vi "SVXMPL_Snd Read Waveform.vi"(8 "error in (no error)":errorcluster, 11 "wave file path":path) -> (0 "error out":errorcluster, 2 "Channel 2":waveform(dbl), 3 "Channel 1":waveform(dbl), 4 "SVT Wav info":T1)   [LabVIEW 2017]
panel:
  in  "SVT Wav info":T1
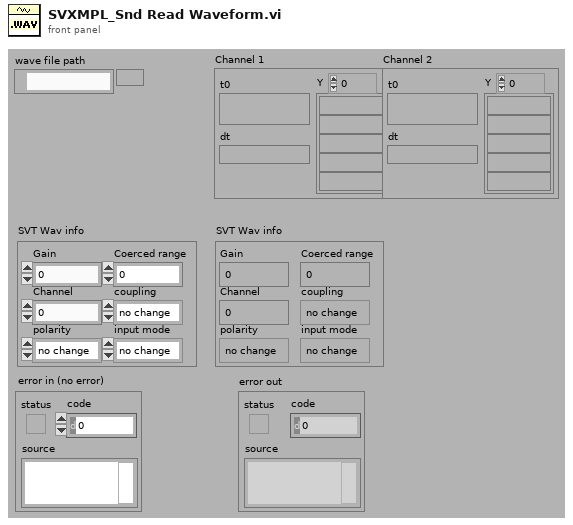
[diagram p1: front panel]
types:
  T1 = cluster{"Gain":u16, "Coerced range":u16, "Channel":u16, "coupling":enum16{"no change", "DC", "AC", "ground", "internal reference"}, "polarity":enum16{"no change", "bipolar", "unipolar"}, "input mode":enum16{"no change", "differential", "rse", "nrse"}}
  T2 = typedef "Sound Format.ctl" = cluster{"sound quality":enum16{"mono", "stereo"}, "rate":enum16{"11025", "22050", "44100", "8000"}, "bits per sample":enum16{"8 bit", "16 bit"}}
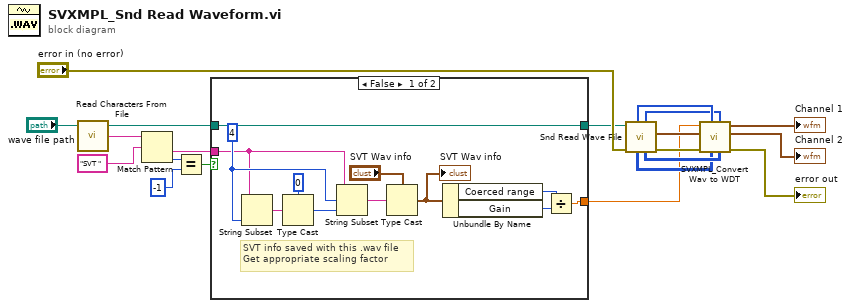
[diagram p0: block diagram]
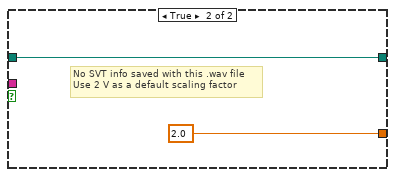
[diagram p2: hidden frame]
diagram:
  n1 = call <vilib>:"Read Characters From File.vi"("file path (dialog if empty)"="wave file path") -> ("new file path (NotAPath if cancelled)"=w5:path, "character string"=w9:string)  [unwired: 5 in, 2 out]
  n2 = Match Pattern(string=w9, regular expression="SVT ") -> (after substring=w2:string, offset past match=w7:i32)  [unwired: 1 in, 2 out]
  n3 = Equal?(x=w7, y=-1) -> (x = y?=w3:bool)
  n4 = case shown="False" w3 {
    tunnel: w5 -> [w32 w34]
    tunnel: [w32 w34] -> w4
    tunnel: w2 -> [w28 _]
    tunnel: [w23 2.0] -> w1
    frame False {
      w31 = 4 ("length (rest)")
      (unwired) 4 ("Array Length")
      # "SVT info saved with this .wav file\nGet appropriate scaling factor"
      n5 = String Subset(string=w28, length (rest)=w31) -> (substring=w30:string)  [unwired: 1 in]
      n6 = Type Cast(type=u32 0, x=w30) -> (*(type *) &x=w27:u32)
      n7 = String Subset(string=w28, offset (0)=w31, length (rest)=w27) -> (substring=w25:string)
      n8 = Type Cast(type="SVT Wav info", x=w25) -> (*(type *) &x=w24:T1)
      "SVT Wav info" <- w24
      n9 = Unbundle By Name(w24) -> ("Coerced range"=w22:u16, "Gain"=w21:u16)
      n10 = Divide(x=w22, y=w21) -> (x/y=w23:dbl)
    }
    frame True {
      # "No SVT info saved with this .wav file\nUse 2 V as a default scaling factor"
    }
  }
  n11 = call <vilib>:"Snd Read Wave File.vi"("error in (no error)"="error in (no error)", "wave file path"=w4) -> ("error out"=w20:errorcluster, "sound format"=w19:T2, "stereo 16-bit"=w15:i16[][], "mono 16-bit"=w17:i16[], "stereo 8-bit"=w14:u8[][], "mono 8-bit"=w18:u8[])  [unwired: 3 in, 1 out]
  n12 = call <vilib>:"SVXMPL_Convert Wav to WDT.vi"("stereo 16-bit"=w15, "mono 16-bit"=w17, "stereo 8-bit"=w14, "mono 8-bit"=w18, "error in (no error)"=w20, "sound format"=w19, "Gain"=w1) -> ("error out"=→"error out":errorcluster, "Channel 2"=→"Channel 2":waveform(dbl), "Channel 1"=→"Channel 1":waveform(dbl))  [unwired: 2 in]
